vi "Rename temporary PDF file.vi"(0 "File path":path, 7 "Temporary File Name":path, 11 "error in (no error)":errorcluster, 12 "Action":enum16{"Delete", "Rename"}(ring)) -> (4 "Duplicate File path":path, 6 "Temporary file path":path, 15 "error out":errorcluster)   [LabVIEW 2019]
doc: "Version 1.0\nDeveloped by Jean-Marc Simard\nCopyright © 2010, Exaprom Inc.\nAll rights reserved.\nLicense: BSD"
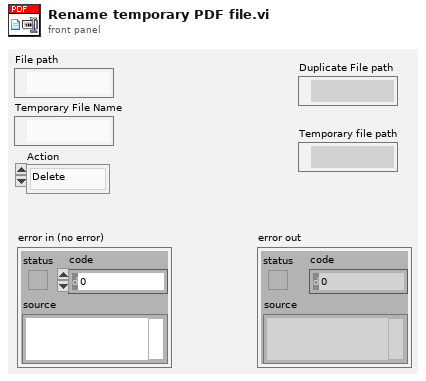
[diagram p1: front panel]
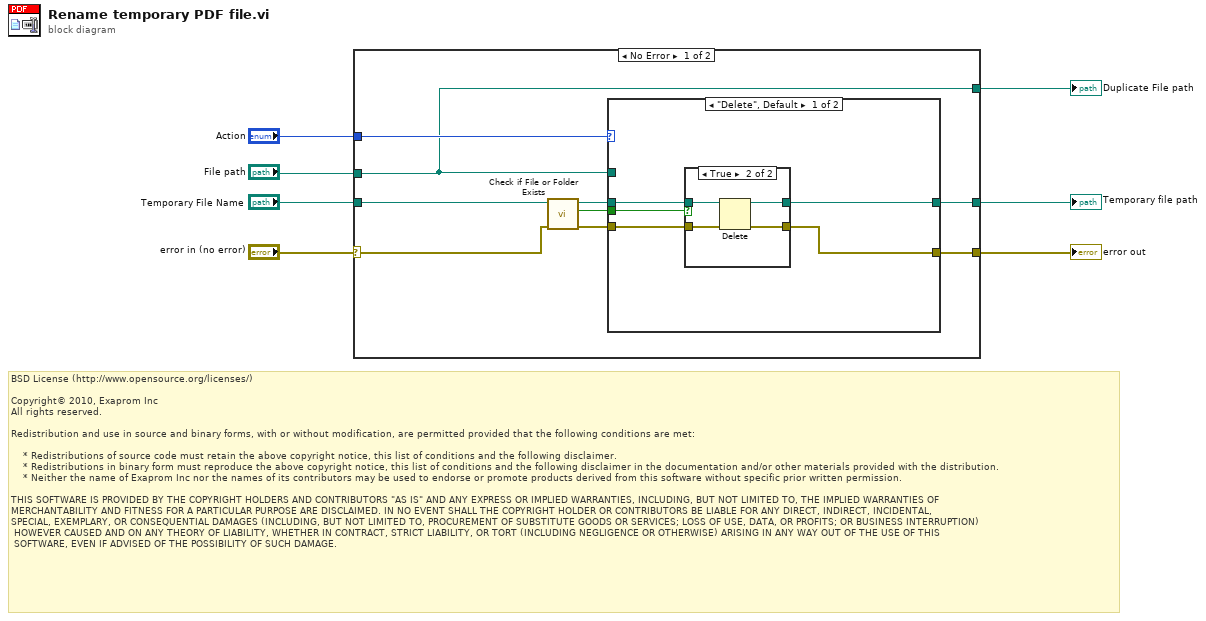
[diagram p0: block diagram]
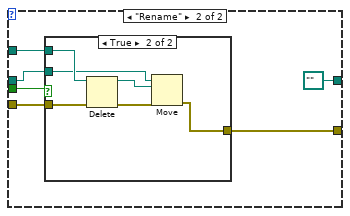
[diagram p3: hidden frame]
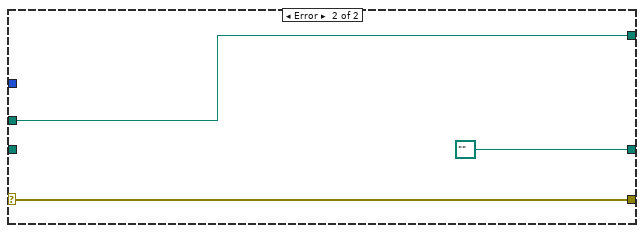
[diagram p5: hidden frame]
diagram:
  # "BSD License (http://www.opensource.org/licenses/)\n\nCopyright© 2010, Exaprom Inc\nAll rights reserved.\n\nRedistribution and use in source and binary forms, with or without modification, are permitted provided that the following conditions are met:\n\n    * Redistributions of source code must retain the above copyright notice, this list of conditions and the following disclaimer.\n    * Redistributions in binary form must reproduce the above copyright notice, this list of conditions and the following disclaimer in the documentation and/or other materials provided with the distribution.\n    * Neither the name of Exaprom Inc nor the names of its contributors may be used to endorse or promote products derived from this software without specific prior written permission.\n\nTHIS SOFTWARE IS PROVIDED BY THE COPYRIGHT HOLDERS AND CONTRIBUTORS \"AS IS\" AND ANY EXPRESS OR IMPLIED WARRANTIES, INCLUDING, BUT NOT LIMITED TO, THE IMPLIED WARRANTIES OF \nMERCHANTABILITY AND FITNESS FOR A PARTICULAR PURPOSE ARE DISCLAIMED. IN NO EVENT SHALL THE COPYRIGHT HOLDER OR CONTRIBUTORS BE LIABLE FOR ANY DIRECT, INDIRECT, INCIDENTAL,\nSPECIAL, EXEMPLARY, OR CONSEQUENTIAL DAMAGES (INCLUDING, BUT NOT LIMITED TO, PROCUREMENT OF SUBSTITUTE GOODS OR SERVICES; LOSS OF USE, DATA, OR PROFITS; OR BUSINESS INTERRUPTION)\n HOWEVER CAUSED AND ON ANY THEORY OF LIABILITY, WHETHER IN CONTRACT, STRICT LIABILITY, OR TORT (INCLUDING NEGLIGENCE OR OTHERWISE) ARISING IN ANY WAY OUT OF THE USE OF THIS\n SOFTWARE, EVEN IF ADVISED OF THE POSSIBILITY OF SUCH DAMAGE."
  n1 = case shown="No Error" "error in (no error)" {
    selector: "error in (no error)" -> [w14 w43]
    tunnel: [w12 w43] -> w6
    tunnel: "File path" -> [w9 w42]
    tunnel: [w11 path "" ("deleted path")] -> w5
    tunnel: [w9 w42] -> w3
    tunnel: "Action" -> [w10 _]
    tunnel: "Temporary File Name" -> [w8 _]
    frame No Error {
      n2 = call <vilib>:"Check if File or Folder Exists.vi"("error in (no error)"=w14, "path"=w8) -> ("error out"=w13:errorcluster, "file or folder exists?"=w16:bool, "dup path"=w15:path)  [unwired: 7 out]
      n3 = case shown="\"Delete\", Default" w10 {
        tunnel: w16 -> [w21 w33]
        tunnel: w15 -> [w20 w30]
        tunnel: w13 -> [w19 w31]
        tunnel: [w18 w29] -> w12
        tunnel: [w17 path "" ("deleted path")] -> w11
        tunnel: w9 -> [_ w32]
        frame "Delete", Default {
          n4 = case shown="True" w21 {
            tunnel: w20 -> [w23 w27]
            tunnel: [w23 w26] -> w17
            tunnel: w19 -> [w22 w25]
            tunnel: [w22 w24] -> w18
            frame False {
            }
            frame True {
              n5 = Delete(path (use dialog)=w27, error in=w25) -> (deleted path=w26:path, error out=w24:errorcluster)  [unwired: 4 out]
            }
          }
        }
        frame "Rename" {
          n6 = case shown="True" w33 {
            tunnel: w32 -> [_ w40]
            tunnel: w31 -> [w34 w39]
            tunnel: w30 -> [_ w37]
            tunnel: [w34 w35] -> w29
            frame False {
            }
            frame True {
              n7 = Delete(path (use dialog)=w40, error in=w39) -> (deleted path=w36:path, error out=w38:errorcluster)  [unwired: 4 out]
              n8 = Move(source path=w37, error in=w38, 10:w36) -> (error out=w35:errorcluster)  [unwired: 4 out]
            }
          }
        }
      }
    }
    frame Error {
    }
  }
  "error out" <- w6
  "Temporary file path" <- w5
  "Duplicate File path" <- w3
